vi "main.vi"   [LabVIEW 2024]
panel:
  # "PolyTheremin \nMeasurement App"
  # "Dependences required: Python v3.10.0"
  # "Milosz Derzko"
types:
  T1 = typedef "#CoreQueues.ctl" = cluster{"DacData":refnum<queue>, "CorrelationData":refnum<queue>, "VideoData":refnum<queue>, "error out":errorcluster, "ToGUI":refnum<queue>, "FileData":refnum<queue>}
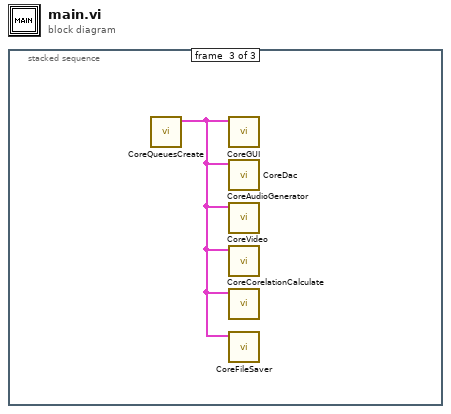
[diagram p0: block diagram]
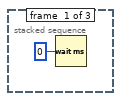
[diagram p2: hidden frame]
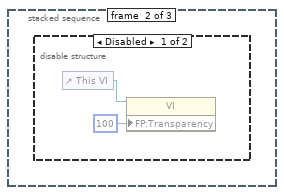
[diagram p3: hidden frame]
diagram:
  n1 = stacked-sequence {
    frame #0 {
      n2 = Wait (ms)(milliseconds to wait=u32 0) -> ()  [unwired: 1 out]
    }
    frame #1 {
      n3 = disable-structure shown="Disabled" {
        frame Disabled {
          n4 = control-ref of="This VI"() -> (w2:refnum<vi>)
          n5 = property class="VI"(reference=w2, "FP:Transparency"=u8 100 ("Front Panel Window:Transparency")) -> ()  [unwired: 1 in, 2 out]
        }
        frame Enabled {
        }
      }
    }
    frame #2 {
      n6 = call "CoreQueuesCreate.vi"() -> ("Cluster"=w4:T1)  [unwired: 11 in]
      n7 = call "CoreGUI.vi"("Cluster"=w4) -> ()  [unwired: 11 in]
      n8 = call "CoreDac.vi"("Cluster"=w4) -> ()  [unwired: 11 in]
      n9 = call "CoreAudioGenerator.vi"("Cluster"=w4) -> ()  [unwired: 11 in]
      n10 = call "CoreVideo.vi"("Cluster"=w4) -> ()  [unwired: 11 in]
      n11 = call "CoreCorelationCalculate.vi"("Cluster"=w4) -> ()  [unwired: 11 in]
      n12 = call "CoreFileSaver.vi"("Cluster"=w4) -> ()  [unwired: 11 in]
    }
  }
